vi "Get Variable Alias.vi"(10 "Variable Name":string, 11 "Device Name":string) -> (3 "Alias":string)   [LabVIEW 2013]
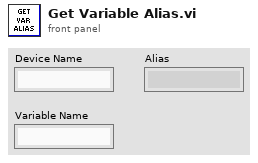
[diagram p1: front panel]
types:
  T1 = typedef "mysql_authentication.ctl" = cluster{"User":string, "Password":string, "Database":string}
  T2 = cluster{"Port":u16, "IP Address":string, "Authentication":T1}
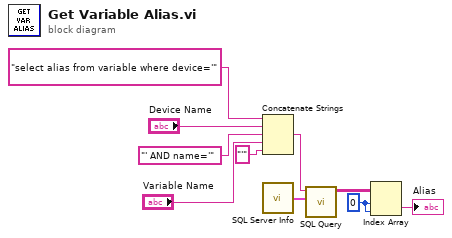
[diagram p0: block diagram]
diagram:
  w9 = 0 ("disabled index (col)")
  n1 = Concatenate Strings("select alias from variable where device='" ("Query"), "Device Name", "' AND name='" ("string"), "Variable Name", "'" ("string")) -> (w1:string)
  n2 = call "SQL Server Info.vi"() -> ("SQL Server Info"=w10:T2)
  n3 = call "SQL Query.vi"("SQL Server Info"=w10, "Query"=w1) -> ("data"=w4:string[][])  [unwired: 8 in, 1 out]
  n4 = Index Array(array=w4, index (row)=w9, index (col)=w9) -> (element=→"Alias":string)
